vi "Abadines_ServerA.vi"() -> ()   [LabVIEW 2013]
uses:
  <vilib>/NXT/Dual Mode Library/Display/drawText.vi
  <vilib>/NXT/Block Support/NXT_InputPort.ctl
  <vilib>/NXT/Dual Mode Library/BT/BlueTooth_Write_String.vi
  <vilib>/NXT/Block Support/NXT_MessageMailbox.ctl
  <vilib>/NXT/Subs/MotorOutput.ctl
panel:
  out "Blue Line":i16
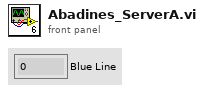
[diagram p1: front panel]
types:
  T1 = typedef "LVHSConnector.ctl" = refnum<class "BrickReference.lvclass">
  T2 = typedef "NXT_InputPort.ctl" = u32
  T3 = typedef "MotorOutput.ctl" = u8
  T4 = typedef "NXT_MessageMailbox.ctl" = u8
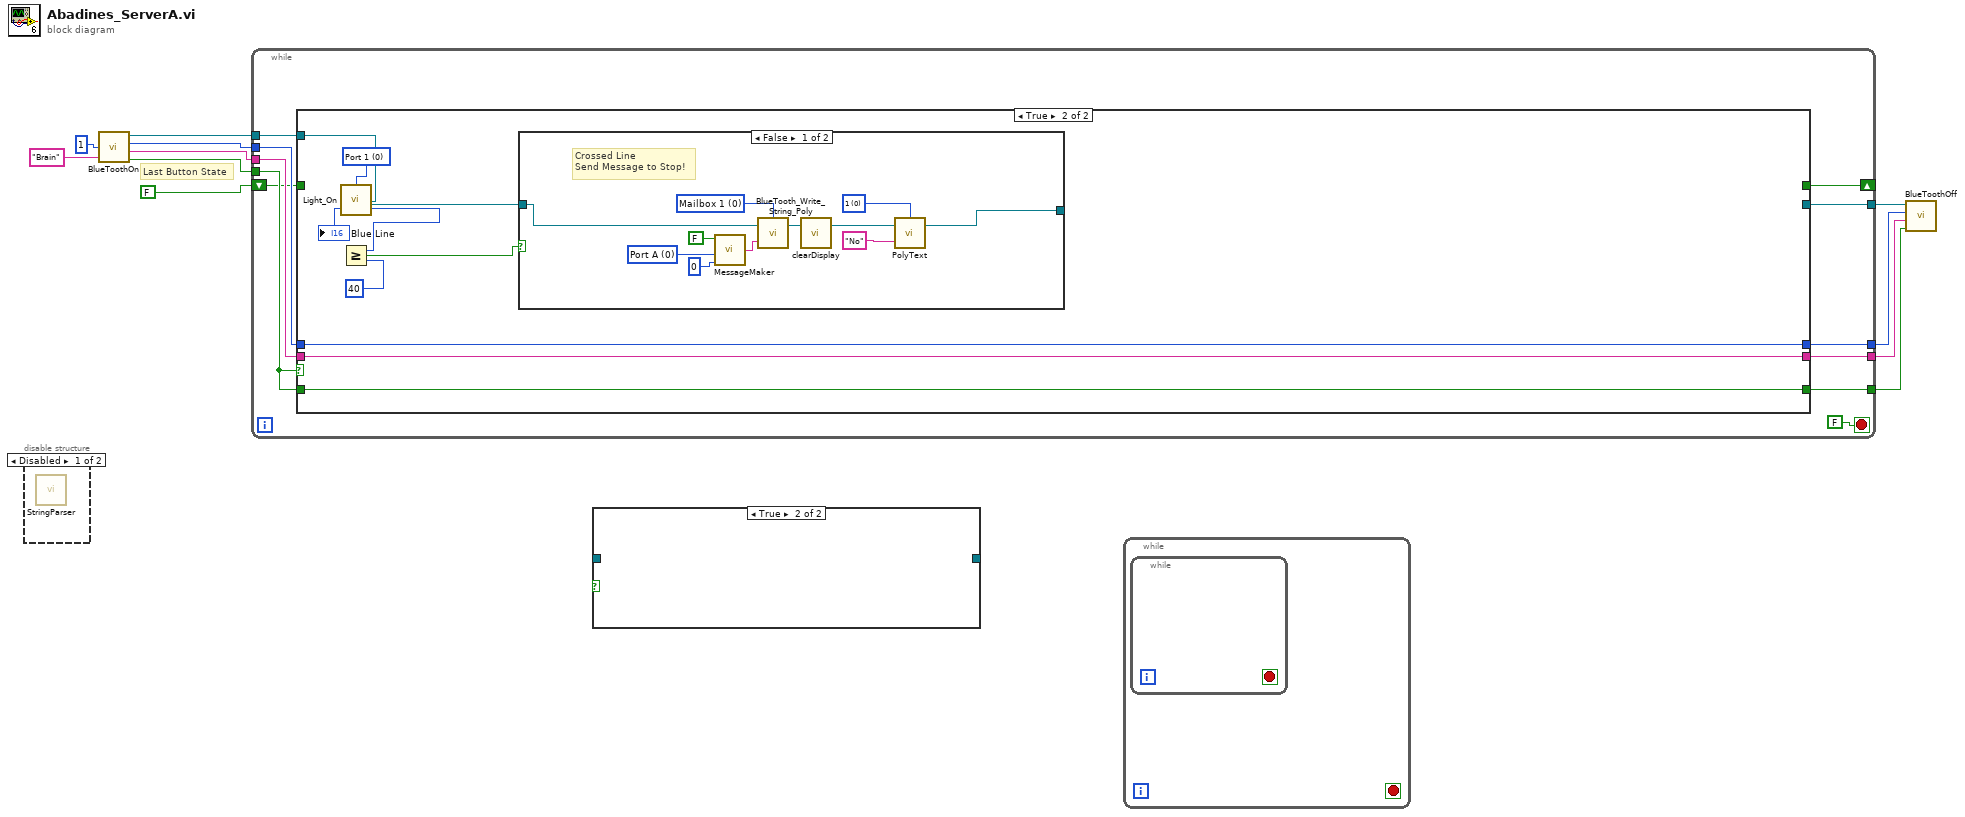
[diagram p0: block diagram]
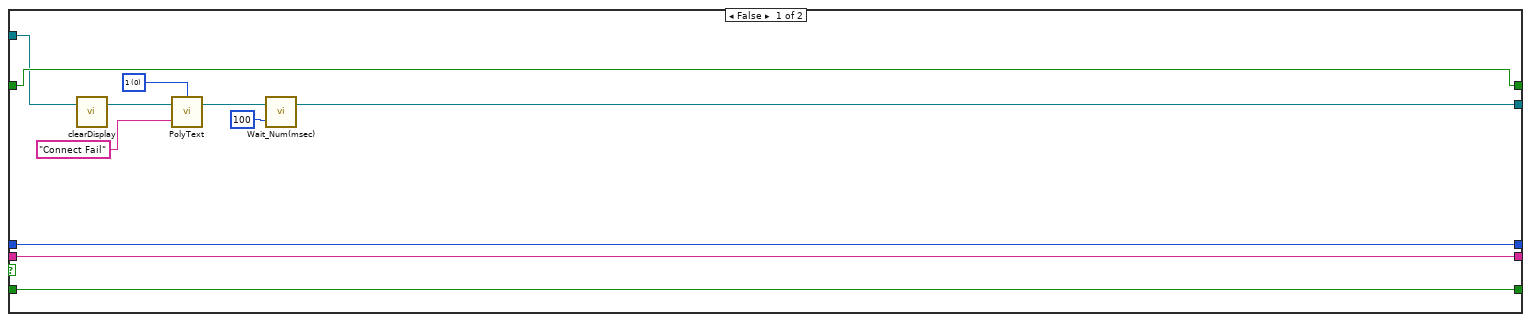
[diagram p3: hidden frame]
diagram:
  # "Last Button State"
  n1 = disable-structure shown="Disabled" {
    frame Disabled {
      n2 = call "StringParser.vi"() -> ()  [unwired: 1 in, 4 out]
    }
    frame Enabled {
    }
  }
  n3 = call "BlueToothOn.vi"("Connection"=u8 1, "Partner Name"="Brain") -> ("NXT/EV3 2"=w9:T1, "Connection"=w8:u8, "Partner Name"=w7:string, "Success"=w6:bool)  [unwired: 1 in]
  n4 = while {
    tunnel: w9 -> [w22]
    tunnel: w8 -> [w21]
    tunnel: w7 -> [w20]
    tunnel: w6 -> [w19]
    tunnel: [w18] -> w5
    tunnel: [w17] -> w4
    tunnel: [w16] -> w3
    tunnel: [w15] -> w2
    shift-right: [w12] -> _
    shift-left: FALSE -> [w13]
    stop <- FALSE stop-if-true
    n5 = case shown="True" w19 {
      tunnel: w22 -> [w28 w39]
      tunnel: w21 -> [w33 w40]
      tunnel: w20 -> [w32 w41]
      tunnel: [w24 _] -> w15
      tunnel: [w33 w40] -> w16
      tunnel: [w32 w41] -> w17
      tunnel: w19 -> [w31 w42]
      tunnel: [w31 w42] -> w18
      tunnel: w13 -> [w30 _]
      tunnel: [w30 _] -> w12
      frame False {
        w27 = i16 0 items=["1", "2", "3", "4", "5", "6", "7", "8", "9", "10", "11", "12"] ("Line")
        n6 = call <vilib>:"clearDisplay.vi"("NXT/EV3"=w28) -> ("NXT/EV3"=w29:T1)  [unwired: 3 in]
        n7 = call-poly <vilib>:"PolyText.vi"("Text"="Connect Fail", "NXT/EV3"=w29, "Line"=w27) -> ("NXT/EV3"=w25:T1)  [unwired: 1 in]
        n8 = call <vilib>:"Wait_Num(msec).vi"("Time (100 msec)"=u32 100, "NXT/EV3"=w25) -> ("NXT/EV3"=w24:T1)  [unwired: 2 in]
      }
      frame True {
        w37 = T2 0 items=["Port 1", "Port 2", "Port 3", "Port 4"] ("Port (Port 3)")
        n9 = call <vilib>:"Light_On.vi"("NXT/EV3"=w39, "Port (Port 3)"=w37) -> ("Scaled Value"=w36:i16, "NXT/EV3"=w38:T1)  [unwired: 1 in]
        "Blue Line" <- w36
        n10 = Greater Or Equal?(x=w36, y=i16 40) -> (x >= y?=w34:bool)
        n11 = case shown="False" w34 {
          tunnel: w38 -> [w44 w54]
          tunnel: [w43 w54] -> _
          frame False {
            w45 = i16 0 items=["1", "2", "3", "4", "5", "6", "7", "8", "9", "10", "11", "12"] ("Line")
            w52 = T3 0 items=["Port A"=0, "Port B"=1, "Port C"=2, "Ports A & B"=4, "Ports A & C"=5, "Ports B & C"=6, "All Ports"=3] ("Output Port (All Ports)")
            w50 = T4 0 items=["Mailbox 1", "Mailbox 2", "Mailbox 3", "Mailbox 4", "Mailbox 5", "Mailbox 6", "Mailbox 7", "Mailbox 8", "Mailbox 9", "Mailbox 10"] ("Mailbox")
            # "Crossed Line\nSend Message to Stop!"
            n12 = call "MessageMaker.vi"("Power"=0, "Output Port (All Ports)"=w52, "R/W (T=R/F=W)"=FALSE) -> ("Message"=w49:string)  [unwired: 1 in]
            n13 = call-poly <vilib>:"BlueTooth_Write_String_Poly.vi"("Message"=w49, "NXT/EV3"=w44, "Mailbox"=w50) -> ("NXT/EV3"=w48:T1)  [unwired: 1 in]
            n14 = call <vilib>:"clearDisplay.vi"("NXT/EV3"=w48) -> ("NXT/EV3"=w47:T1)  [unwired: 3 in]
            n15 = call-poly <vilib>:"PolyText.vi"("Text"="No", "NXT/EV3"=w47, "Line"=w45) -> ("NXT/EV3"=w43:T1)  [unwired: 1 in]
          }
          frame True {
            # "Do Nothing.\nBlue Line Not Crossed"
          }
        }
      }
    }
  }
  n16 = case shown="True" {
    selector: _ -> [_ _]
    tunnel: _ -> [w55 _]
    tunnel: [w55 _] -> _
    frame False {
    }
    frame True {
    }
  }
  n17 = while {
    stop <- _ stop-if-true
    n18 = while {
      stop <- _ stop-if-true
    }
  }
  n19 = call "BlueToothOff.vi"("Connected"=w5, "Partner Name"=w4, "Connection"=w3, "NXT/EV3"=w2) -> ()  [unwired: 1 in, 3 out]
